vi "Update Speed Iteration.vi"(9 "Triggers in":dbl, 11 "Flying Saucer in":refnum<class "Flying Saucer.lvclass">) -> (3 "Flying Saucer out":refnum<class "Flying Saucer.lvclass">)   [LabVIEW 2024, in "Flying Saucer.lvclass"]
doc: "MIT Licence\nCopyright (c) 2024 David Grollier"
uses:
  Flying Saucer.lvclass
  Flying Saucer.lvclass/Flying Saucer.ctl
  Movable.lvclass
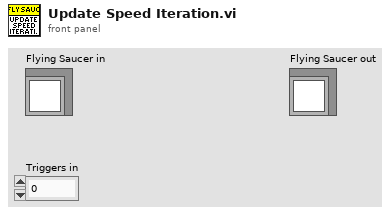
[diagram p1: front panel]
types:
  T1 = typedef "Velocity.ctl" = cluster{"Vx":dbl, "Vy":dbl}
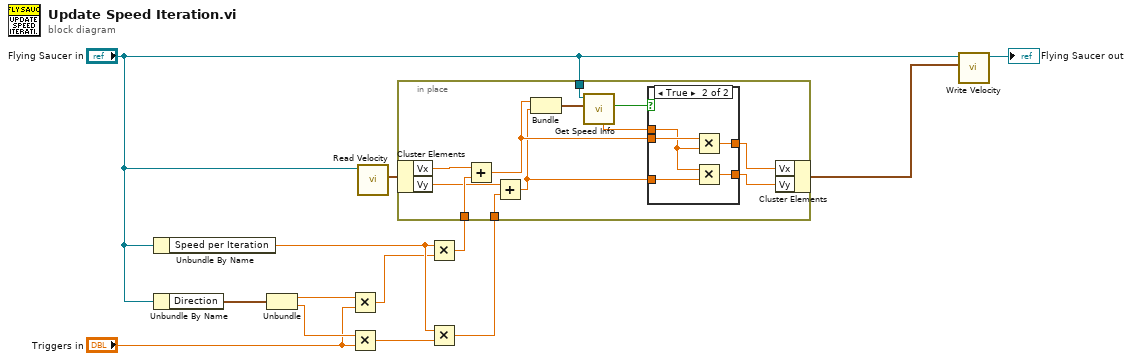
[diagram p0: block diagram]
diagram:
  n1 = Unbundle By Name("Flying Saucer in") -> ("Speed per Iteration"=w10:dbl)
  n2 = Unbundle By Name("Flying Saucer in") -> ("Direction"=w2:T1)
  n3 = Unbundle(w2) -> ("Vx"=w7:dbl, "Vy"=w6:dbl)
  n4 = Multiply(x=w7, y="Triggers in") -> (x*y=w3:dbl)
  n5 = Multiply(x=w6, y="Triggers in") -> (x*y=w4:dbl)
  n6 = call-dynamic "Read Velocity.vi"("Movable in"="Flying Saucer in") -> ("Velocity"=w12:T1)  [unwired: 10 in]
  n7 = Multiply(x=w10, y=w3) -> (x*y=w9:dbl)
  n8 = Multiply(x=w10, y=w4) -> (x*y=w8:dbl)
  n9 = in-place {
    in-place-border: w9 -> [w24]
    in-place-border: w8 -> [w22]
    in-place-border: "Flying Saucer in" -> [w20]
    n10 = in-place-cluster #1(w12) -> ("Vx"=w25:dbl, "Vy"=w23:dbl)
    n11 = Add(x=w25, y=w24) -> (x+y=w19:dbl)
    n12 = Add(x=w23, y=w22) -> (x+y=w18:dbl)
    n13 = Bundle(w19, w18) -> (w21:cluster{dbl, dbl})  [unwired: 1 in]
    n14 = call "Get Speed Info.vi"("Velocity in"=w21, "Movable in"=w20) -> ("Max speed?"=w17:bool, "ratio out"=w16:dbl)  [unwired: 8 in]
    n15 = case shown="True" w17 {
      tunnel: w19 -> [w27 w32]
      tunnel: [w27 w31] -> w15
      tunnel: [w26 w30] -> w14
      tunnel: w18 -> [w26 w29]
      tunnel: w16 -> [_ w28]
      frame False {
      }
      frame True {
        n16 = Multiply(x=w32, y=w28) -> (x*y=w31:dbl)
        n17 = Multiply(x=w28, y=w29) -> (x*y=w30:dbl)
      }
    }
    n18 = in-place-cluster #1("Vx"=w15, "Vy"=w14) -> (w13:T1)
  }
  n19 = call "Write Velocity.vi"("Velocity"=w13, "Movable in"="Flying Saucer in") -> ("Movable out"=→"Flying Saucer out":refnum<class "Flying Saucer.lvclass">)  [unwired: 9 in]
